vi "WriteByteInUART.vi"(7 "error  in":errorcluster, 9 "Byte Value":u8, 10 "FPGA VI Reference In":refnum<k20>) -> (0 "error out":errorcluster, 2 "Overflow?":bool, 3 "FPGA VI Reference Out":refnum<k20>)   [LabVIEW 2016]
uses:
  <vilib>/Utility/error.llb/Error Cluster From Error Code.vi
  <vilib>/rvi/errors/niLvFpgaAdjustHostInterfaceError.vi
  <vilib>/rvi/interface/nirviReadWriteControl/nirviReadWriteControl.xnode
  <vilib>/rvi/interface/Simulation/niFpgaSimulationCallBeginRW.vi
  NiFpgaLv.dll
panel:
  out "millisec":u32
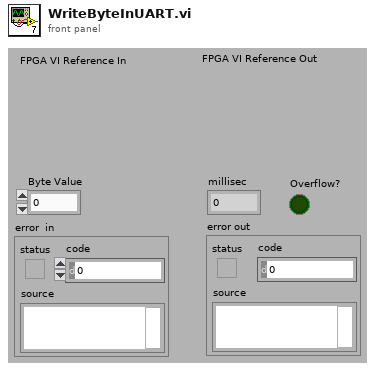
[diagram p1: front panel]
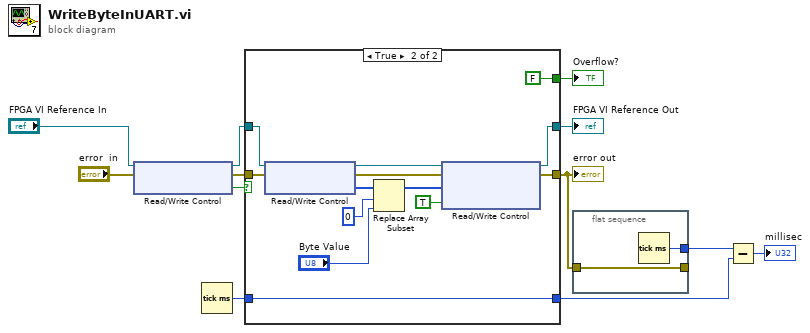
[diagram p0: block diagram]
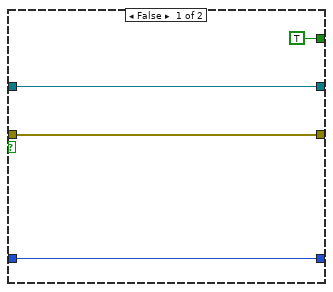
[diagram p2: hidden frame]
diagram:
  n1 = xnode "Read/Write Control"("FPGA VI Reference In"="FPGA VI Reference In", "error in"="error  in") -> ("FPGA VI Reference Out"=w12:refnum<k20>, "error out"=w11:errorcluster, "UART.Tx Ready"=w10:bool)
  n2 = Tick Count (ms)() -> (millisecond timer value=w5:u32)
  n3 = case shown="True" w10 {
    tunnel: w12 -> [w16 w29]
    tunnel: w11 -> [w15 w28]
    tunnel: [w16 w21] -> w1
    tunnel: [w15 w20] -> w3
    tunnel: [TRUE ("Overflow?") FALSE ("Overflow?")] -> w9
    tunnel: w5 -> [w13 w18]
    tunnel: [w13 w18] -> w8
    frame False {
    }
    frame True {
      n4 = xnode "Read/Write Control"("FPGA VI Reference In"=w29, "error in"=w28) -> ("FPGA VI Reference Out"=w23:refnum<k20>, "error out"=w22:errorcluster, "UART.Tx Data"=w17:u8[])
      n5 = Replace Array Subset(array=w17, new element="Byte Value", index=i8 0) -> (w25:u8[])
      n6 = xnode "Read/Write Control"("FPGA VI Reference In"=w23, "error in"=w22, "UART.Tx Data"=w25, "UART.Transmit"=TRUE ("Send Command")) -> ("FPGA VI Reference Out"=w21:refnum<k20>, "error out"=w20:errorcluster)
    }
  }
  "Overflow?" <- w9
  "error out" <- w3
  "FPGA VI Reference Out" <- w1
  n7 = flat-sequence {
    tunnel: [w31] -> w7
    tunnel: [w30] -> _
    tunnel: w3 -> [w30]
    frame #0 {
      n8 = Tick Count (ms)() -> (millisecond timer value=w31:u32)
    }
  }
  n9 = Subtract(x=w7, y=w8) -> (x-y=→"millisec":u32)
